vi "Amira Bladder Experiment V1.0.vi"() -> ()   [LabVIEW 2020]
uses:
  <userlib>/KQD LabVIEW User/Serial/Controls/SERIAL PortConfig.ctl
  <userlib>/KQD LabVIEW User/Serial/Controls/SERIAL BaudRate.ctl
  <userlib>/Amira UART/Public/TypeDefs/AUART StepDir.ctl
  <userlib>/Amira UART/Amira UART.lvclass
  <userlib>/KQD LabVIEW User/Serial/Serial.lvlib
panel:
  in  "RunWith":cluster{"Steps":i32, "Rates":i32}={"Steps"=400, "Rates"=40}
  in  "Folder":path=path "C:/Amira Data/Strip"
  in  "Strip":enum16{"Surface", "Blader"}(ring)
  out "FrontOpen":dbl
  out "BackOpen":dbl
  out "FrontClose":dbl
  out "BackClose":dbl
  in  "StartAt":cluster{"Steps":i32, "Rates":i32}={"Steps"=950, "Rates"=200}
  out "Position":dbl[](graph)
  in  "DAQ":tag="Dev1/port0"
  out "UART":string
  in  "ComPort":refnum<visa-resource-name>
  in  "Config":T1={"BaudRate"=enum."460800", "StopBits"=10, "DataBits"=8, "Parity"=enum."None", "FlowControl"=2, "TimeOut"=1000, "TermChar"=10, "ReadTermEn"=TRUE} {"TermChar" format="%.0x"; "FlowControl" items=["None", "XON/XOFF", "RTS/CTS", "XON/XOFF & RTS/CTS", "DTR/DSR", "XON/XOFF & DTR/DSR"]; "DataBits" min=5 max=8 step=1; "StopBits" items=["1.0"=10, "1.5"=15, "2.0"=20]}
  out "ErrOut":errorcluster
  in  "ErrIn":errorcluster
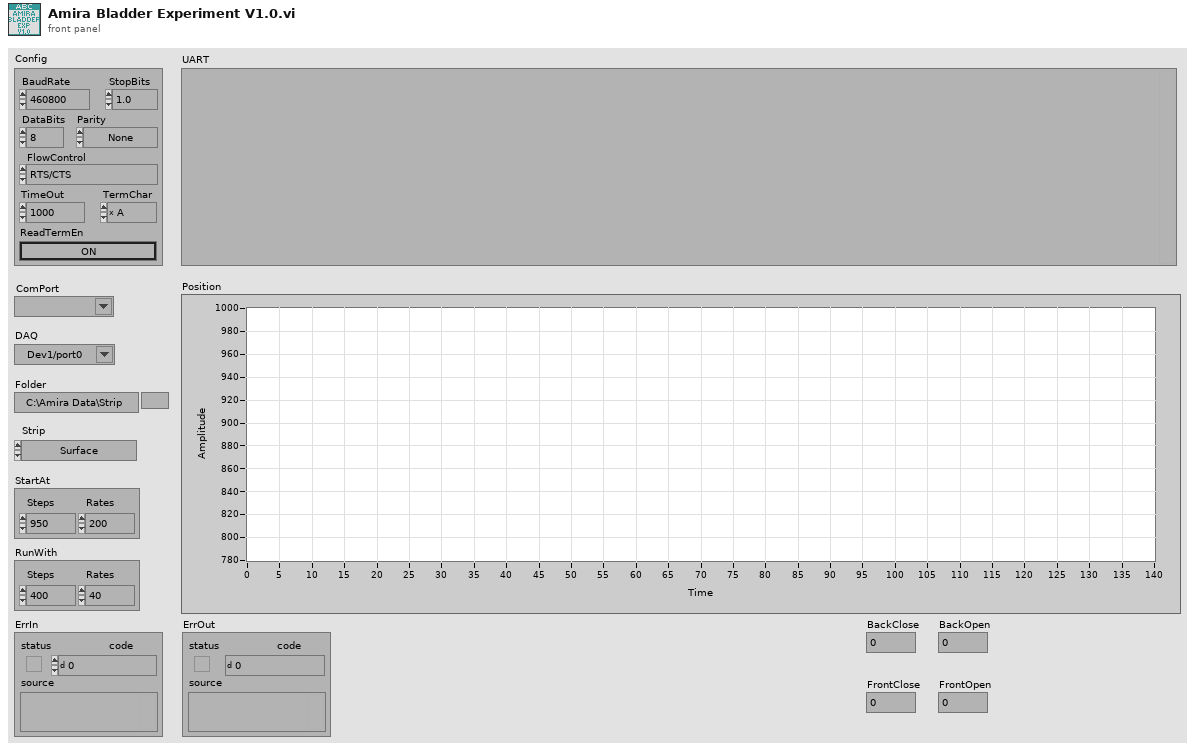
[diagram p1: front panel]
types:
  T1 = typedef "Serial.lvlib/SERIAL PortConfig.ctl" = cluster{"BaudRate":T2, "StopBits":u16, "DataBits":u16, "Parity":enum16{"None", "Odd", "Even", "Mark", "Space"}, "FlowControl":u16, "TimeOut":u32, "TermChar":u8, "ReadTermEn":bool}
  T2 = typedef "SERIAL BaudRate.ctl" = enum16{"2400", "4800", "7200", "9600", "14400", "19200", "28800", "38400", "57600", "115200", "128000", "230400", "460800", "921600"}
  T3 = typedef "Amira UART.lvclass/AUART StepDir.ctl" = enum16{"", "compress", "decompress"}
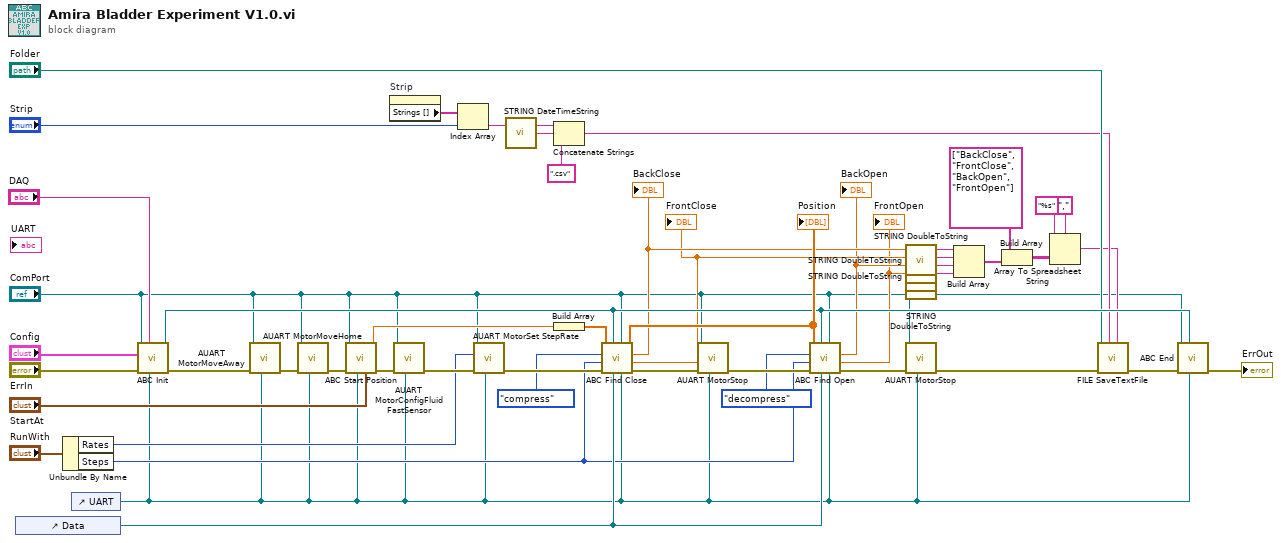
[diagram p0: block diagram]
diagram:
  n1 = control-ref of="Data"() -> (w34:refnum<vi>)
  n2 = Unbundle By Name("RunWith") -> ("Rates"=w9:i32, "Steps"=w8:i32)
  n3 = control-ref of="UART"() -> (w5:refnum<vi>)
  n4 = call "ABC Init.vi"("UART"=w5, "DAQ"="DAQ", "ErrIn"="ErrIn", "PortConfig"="Config", "ComPort"="ComPort") -> ("ErrOut"=w7:errorcluster, "DaqTask"=w35:refnum<k21>)  [unwired: 5 in]
  n5 = call <userlib>:"AUART MotorMoveAway.vi"("UART"=w5, "ErrIn"=w7, "Port"="ComPort") -> ("ErrOut"=w6:errorcluster)  [unwired: 8 in]
  n6 = call <userlib>:"AUART MotorMoveHome.vi"("UART"=w5, "ErrIn"=w6, "Port"="ComPort") -> ("ErrOut"=w45:errorcluster)  [unwired: 7 in, 1 out]
  n7 = call "ABC Start Position.vi"("Start"="StartAt", "UART"=w5, "ErrIn"=w45, "ComPort"="ComPort") -> ("ErrOut"=w44:errorcluster, "LastPos"=w41:dbl)  [unwired: 6 in]
  n8 = property on="Strip" class="Enum (strict)"() -> ("Strings []"=w29:string[])  [unwired: 2 in, 2 out]
  n9 = call <userlib>:"AUART MotorConfigFluidFastSensor.vi"("UART"=w5, "ErrIn"=w44, "Port"="ComPort") -> ("ErrOut"=w47:errorcluster)  [unwired: 8 in]
  n10 = Index Array(array=w29, index="Strip") -> (element=w27:string)
  n11 = call <userlib>:"AUART MotorSet StepRate.vi"("UART"=w5, "ErrIn"=w47, "step_rate"=w9, "Port"="ComPort") -> ("ErrOut"=w46:errorcluster)  [unwired: 7 in]
  n12 = call <userlib>:"STRING DateTimeString.vi"() -> ("DateTimeStr"=w26:string)  [unwired: 2 in]
  n13 = Concatenate Strings(w27, w26, ".csv" ("string")) -> (w23:string)
  n14 = Build Array(w41) -> (w42:dbl[])
  n15 = call "ABC Find Close.vi"("UART"=w5, "ComPort"="ComPort", "Data"=w34, "DaqTask"=w35, "ErrIn"=w46, "#Step"=w8, "Dir"=AUART_StepDir."compress" ("step_dir"), "DataIn"=w42) -> ("ErrOut"=w39:errorcluster, "FrontClose"=w32:dbl, "BackClose"=w33:dbl, "DataOut"=w36:dbl[])
  "Position" <- w36
  "BackClose" <- w33
  "FrontClose" <- w32
  n16 = call <userlib>:"AUART MotorStop.vi"("UART"=w5, "ErrIn"=w39, "Port"="ComPort") -> ("ErrOut"=w38:errorcluster)  [unwired: 8 in]
  n17 = call "ABC Find Open.vi"("UART"=w5, "ComPort"="ComPort", "Data"=w34, "DaqTask"=w35, "ErrIn"=w38, "#Step"=w8, "Dir"=AUART_StepDir."decompress" ("step_dir"), "DataIn"=w36) -> ("ErrOut"=w37:errorcluster, "FrontOpen"=w30:dbl, "BackOpen"=w31:dbl)  [unwired: 1 out]
  "BackOpen" <- w31
  "FrontOpen" <- w30
  n18 = call <userlib>:"STRING DoubleToString.vi"("Num"=w33) -> ("DblStr"=w22:string)  [unwired: 3 in]
  n19 = call <userlib>:"STRING DoubleToString.vi"("Num"=w32) -> ("DblStr"=w21:string)  [unwired: 3 in]
  n20 = call <userlib>:"STRING DoubleToString.vi"("Num"=w31) -> ("DblStr"=w20:string)  [unwired: 3 in]
  n21 = call <userlib>:"STRING DoubleToString.vi"("Num"=w30) -> ("DblStr"=w19:string)  [unwired: 3 in]
  n22 = call <userlib>:"AUART MotorStop.vi"("UART"=w5, "ErrIn"=w37, "Port"="ComPort") -> ("ErrOut"=w3:errorcluster)  [unwired: 8 in]
  n23 = Build Array(w22, w21, w20, w19) -> (w17:string[])
  n24 = Build Array(string[] ["BackClose", "FrontClose", "BackOpen", "FrontOpen"], w17) -> (w16:string[][])
  n25 = Array To Spreadsheet String(delimiter (Tab)=",", array=w16, 3:"%s" ("format string")) -> (spreadsheet string=w14:string)
  n26 = call <userlib>:"FILE SaveTextFile.vi"("Data"=w14, "File"=w23, "ErrIn"=w3, "Folder"="Folder") -> ("ErrOut"=w2:errorcluster)  [unwired: 7 in]
  n27 = call "ABC End.vi"("UART"=w5, "DaqTask"=w35, "ErrIn"=w2, "ComPort"="ComPort") -> ("ErrOut"=→"ErrOut":errorcluster)  [unwired: 7 in]
